vi "Test Process Throws Error on Invalid Name.vi"(8 "error in (no error)":errorcluster, 11 "Process Test in":refnum<class "Process Test.lvclass">) -> (0 "error out":errorcluster, 3 "Process Test out":refnum<class "Process Test.lvclass">)   [LabVIEW 2020, in "Process Test.lvclass"]
uses:
  Process Test.lvclass
  Process Test.lvclass/Process Test.ctl
  Framework/Process/Process.lvclass
  <vilib>/Astemes/LUnit/Test Case.lvclass
  C:/Git/astemes-triarc-framework/source/Framework Test/Base Class Test/Base Test.lvclass
  C:/Program Files (x86)/National Instruments/LabVIEW 2020/vi.lib/Astemes/LUnit/Test Case.lvclass
  C:/Git/astemes-triarc-framework/source/Framework Test/Process Test/Process Test.lvclass
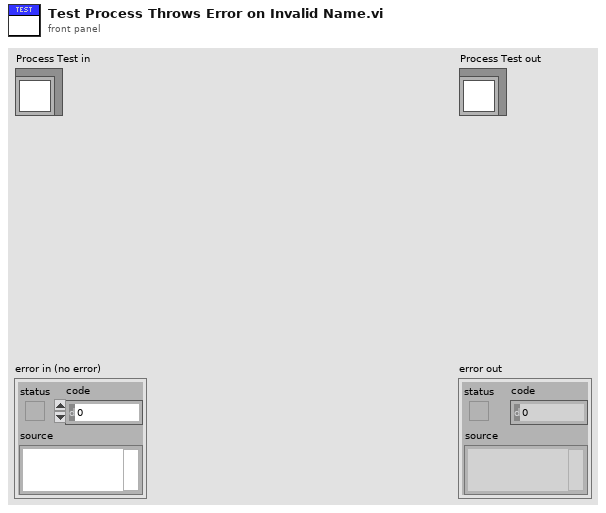
[diagram p1: front panel]
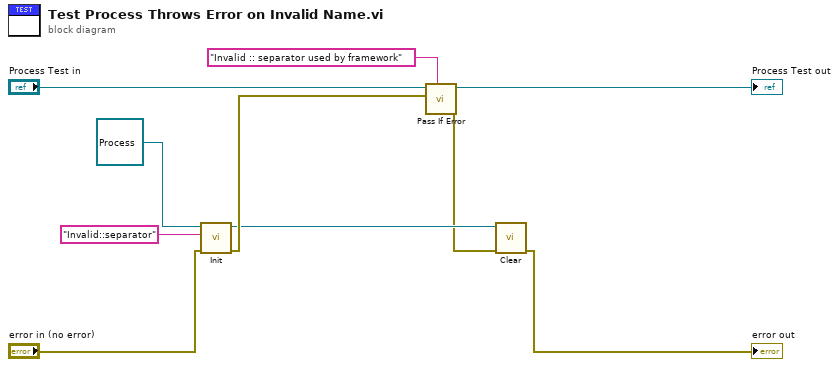
[diagram p0: block diagram]
diagram:
  n1 = call-dynamic "Init.vi"("error in (no error)"="error in (no error)", "Name"="Invalid::separator", "Process In"=refnum<class "Process.lvclass"> refnum) -> ("error out"=w7:errorcluster, "Process Out"=w3:refnum<class "Process.lvclass">)  [unwired: 7 in]
  n2 = call <vilib>:"Pass If Error.vi"("Description"="Invalid :: separator used by framework", "Assert error"=w7, "LUnit Test Case In"="Process Test in") -> ("error out"=w2:errorcluster, "LUnit Test Case Out"=→"Process Test out":refnum<class "Process Test.lvclass">)  [unwired: 7 in]
  n3 = call-dynamic "Clear.vi"("error in (no error)"=w2, "Process In"=w3) -> ("error out"=→"error out":errorcluster)  [unwired: 9 in]
